vi "Memory.Pointer.Deallocate.vi"(8 "error in (no error)":errorcluster, 11 "Pointer in":refnum<class "Memory.Pointer.lvclass">) -> (0 "error out":errorcluster, 3 "Pointer out":refnum<class "Memory.Pointer.lvclass">)   [LabVIEW 2016, in "Memory Manager.lvlib" / "Memory.Pointer.lvclass"]
uses:
  Memory.Pointer.lvclass
  Memory.Pointer.Errors.Zone.vi
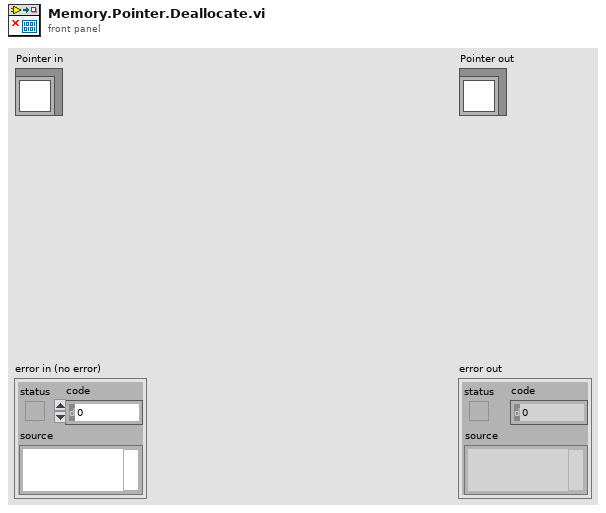
[diagram p1: front panel]
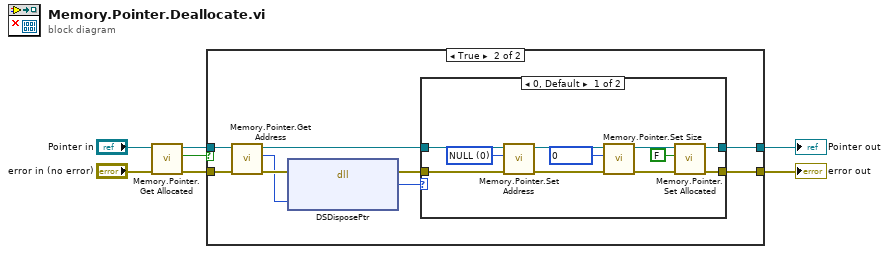
[diagram p0: block diagram]
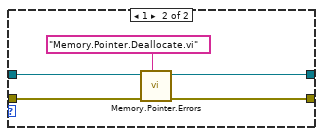
[diagram p3: hidden frame]
diagram:
  n1 = call "Memory.Pointer.Get Allocated.vi"("Pointer in"="Pointer in") -> ("allocated"=w2:bool, "Pointer out"=w3:refnum<class "Memory.Pointer.lvclass">)  [unwired: 9 in]
  n2 = case shown="True" w2 {
    tunnel: [w8 w16] -> w6
    tunnel: [w7 w15] -> w5
    tunnel: w3 -> [w8 w12]
    tunnel: "error in (no error)" -> [w7 w10]
    frame False {
    }
    frame True {
      n3 = call "Memory.Pointer.Get Address.vi"("Pointer in"=w12) -> ("address"=w9:u64, "Pointer out"=w11:refnum<class "Memory.Pointer.lvclass">)  [unwired: 9 in]
      n4 = dll-call lib="LabVIEW" fn="DSDisposePtr"(error in=w10, "pointer"=w9) -> (error out=w14:errorcluster, "return"=w13:i32)  [unwired: 3 in, 1 out]
      n5 = case shown="0, Default" w13 {
        tunnel: w14 -> [w20 w29]
        tunnel: [w20 w28] -> w15
        tunnel: [w18 w27] -> w16
        tunnel: w11 -> [w24 w26]
        frame 0, Default {
          w21 = u64 0 items=["NULL"] ("Null")
          n6 = call "Memory.Pointer.Set Address.vi"("address"=w21, "Pointer in"=w24) -> ("Pointer out"=w23:refnum<class "Memory.Pointer.lvclass">)  [unwired: 9 in]
          n7 = call "Memory.Pointer.Set Size.vi"("size"=u64 0, "Pointer in"=w23) -> ("Pointer out"=w19:refnum<class "Memory.Pointer.lvclass">)  [unwired: 9 in]
          n8 = call "Memory.Pointer.Set Allocated.vi"("allocated"=FALSE, "Pointer in"=w19) -> ("Pointer out"=w18:refnum<class "Memory.Pointer.lvclass">)  [unwired: 9 in]
        }
        frame 1 {
          n9 = call-poly "Memory.Pointer.Errors.vi"("error source vi name"="Memory.Pointer.Deallocate.vi" ("source vi name"), "error in (no error)"=w29, "Pointer in"=w26) -> ("error out"=w28:errorcluster, "Pointer out"=w27:refnum<class "Memory.Pointer.lvclass">)  [unwired: 7 in]
        }
      }
    }
  }
  "error out" <- w5
  "Pointer out" <- w6
